vi "Insert Loop.vi"(4 "Loop Iterations":i32, 6 "Insertion Index":i32=-1, 7 "Parent ID":string, 8 "error in (no error)":errorcluster, 9 "Unique ID":string, 10 "Name":string, 11 "Custom Type Test Executive in":refnum<class "Custom Type Test Executive.lvclass">) -> (0 "error out":errorcluster, 1 "Replaced?":bool, 2 "Unique ID out":string, 3 "Custom Type Test Executive out":refnum<class "Custom Type Test Executive.lvclass">)   [LabVIEW 2017, in "Custom Type Test Executive.lvlib" / "Custom Type Test Executive.lvclass"]
uses:
  <vilib>/gpm_packages/@cs/test-executive/Source/Custom Type Test Executive/Custom Type Test Executive/Custom Type Test Executive.lvclass
  C:/Program Files/National Instruments/LabVIEW 2017/vi.lib/gpm_packages/@cs/test-executive/Source/Test Executive/TestExecutive/Test Executive.lvclass
  <vilib>/gpm_packages/@cs/test-executive/Source/Custom Type Test Executive/Loop/Loop.lvclass
  <vilib>/gpm_packages/@cs/data-type-serializer/source/Boolean/Boolean.lvclass/Boolean.ctl
  <vilib>/gpm_packages/@cs/data-type-serializer/source/I32/I32.lvclass/I32.ctl
  <vilib>/gpm_packages/@cs/test-executive/Source/Test Executive/TestExecutive/Test Executive.lvclass/Test Executive.ctl
  eff3c389-d19d-4e12-abfe-b5bcb03aec03.vi
  3b5f5b1c-5d92-47fe-9b34-6cf7948e1255.vi
  2e520cd6-f760-4b31-8e6b-f4272244ae2a.vi
  34c56a90-4072-42ae-b3b1-584153b934c7.vi
  <vilib>/gpm_packages/@cs/data-type-serializer/source/I32/I32.lvclass
  <vilib>/gpm_packages/@cs/data-type-serializer/source/Boolean/Boolean.lvclass
  <vilib>/gpm_packages/@cs/linked-list/Source/Linked List/ILinkedList/ILinked List.lvclass
  <vilib>/gpm_packages/@cs/linked-list/Source/Linked List/Linked List Ref/Linked List Ref.lvclass
  <vilib>/gpm_packages/@cs/test-executive/Source/Test Executive/TestExecutive/Test Executive.lvclass
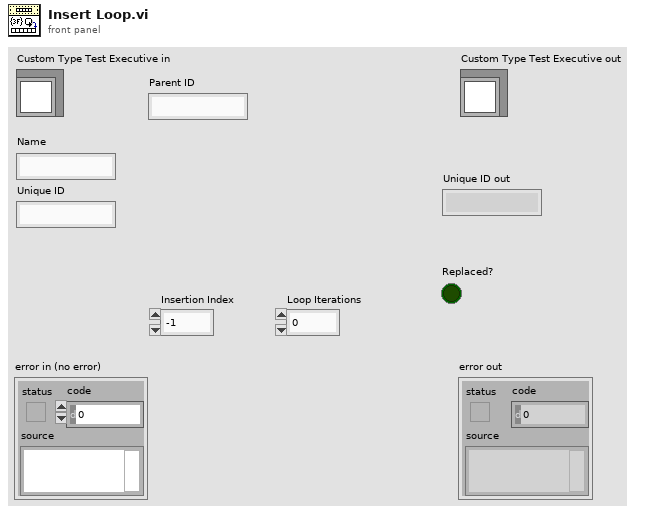
[diagram p1: front panel]
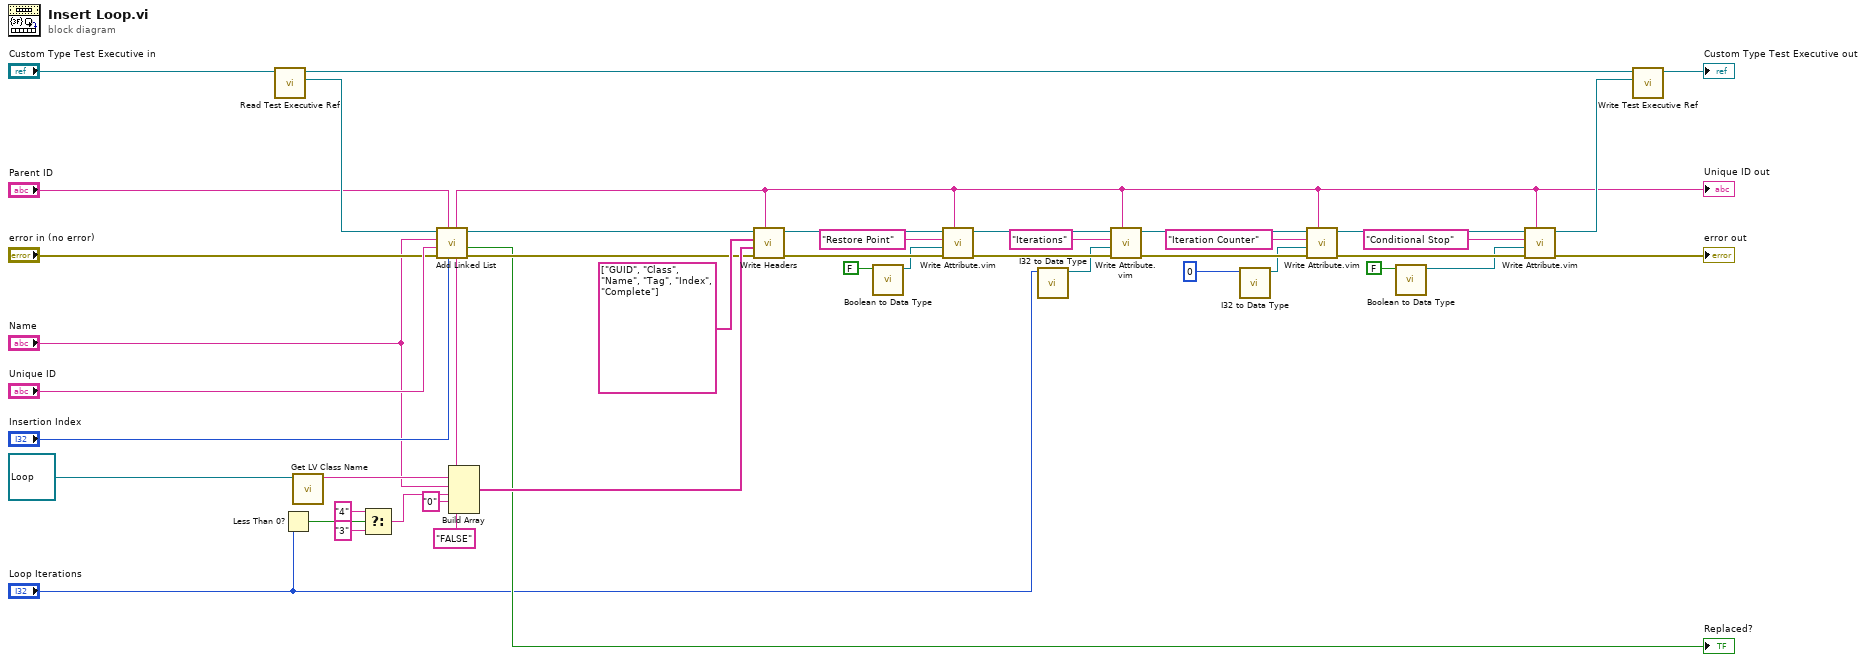
[diagram p0: block diagram]
diagram:
  n1 = call <vilib>:"Read Test Executive Ref.vi"("Test Executive in"="Custom Type Test Executive in") -> ("Test Executive Ref"=w21:refnum<data-value>, "Test Executive out"=w20:refnum<class "Custom Type Test Executive.lvclass">)  [unwired: 9 in]
  n2 = Less Than 0?(x="Loop Iterations") -> (x < 0?=w37:bool)
  n3 = call <vilib>:"Get LV Class Name.vi"("object"=refnum<class "Loop.lvclass"> refnum ("Custom Type Test Executive.lvlib:Loop.lvclass")) -> ("class name"=w41:string)  [unwired: 9 in, 1 out]
  n4 = Select(t="4" ("Tag"), s=w37, f="3" ("Tag")) -> (s? t:f=w34:string)
  n5 = call <vilib>:"Add Linked List.vi"("Insertion Index"="Insertion Index", "Parent ID"="Parent ID", "error in (no error)"="error in (no error)", "Linked List ID"="Unique ID", "Name"="Name", "Linked List Ref"=w21) -> ("error out"=w42:errorcluster, "Replaced?"=→"Replaced?":bool, "Linked List Ref out"=w43:refnum<data-value>, "Linked List ID out"=w12:string)  [unwired: 2 in]
  "Unique ID out" <- w12
  n6 = Build Array(w12, w41, "Name", w34, "0" ("element"), "FALSE" ("element")) -> (w44:string[])
  n7 = call <vilib>:"Write Headers.vi"("Linked List ID"=w12, "error in (no error)"=w42, "Header Values"=w44, "Header Names"=string[] ["GUID", "Class", "Name", "Tag", "Index", "Complete"], "Linked List Ref"=w43) -> ("error out"=w38:errorcluster, "Linked List Ref out"=w39:refnum<data-value>)  [unwired: 5 in]
  n8 = call <vilib>:"Boolean to Data Type.vi"("Boolean"=FALSE) -> ("Boolean out"=w7:refnum<class "Boolean.lvclass">)  [unwired: 9 in, 1 out]
  n9 = call "Write Attribute.vim"("Linked List ID"=w12, "error in (no error)"=w38, "Attribute"=w7, "Attribute Name"="Restore Point", "Linked List Ref"=w39) -> ("error out"=w27:errorcluster, "Linked List Ref out"=w30:refnum<data-value>)  [unwired: 3 in, 2 out]
  n10 = call <vilib>:"I32 to Data Type.vi"("I32"="Loop Iterations") -> ("Boolean out"=w5:refnum<class "I32.lvclass">)  [unwired: 9 in, 1 out]
  n11 = call "Write Attribute.vim"("Linked List ID"=w12, "error in (no error)"=w27, "Attribute"=w5, "Attribute Name"="Iterations", "Linked List Ref"=w30) -> ("error out"=w26:errorcluster, "Linked List Ref out"=w29:refnum<data-value>)  [unwired: 3 in, 2 out]
  n12 = call <vilib>:"I32 to Data Type.vi"("I32"=0 ("Numeric")) -> ("Boolean out"=w3:refnum<class "I32.lvclass">)  [unwired: 9 in, 1 out]
  n13 = call "Write Attribute.vim"("Linked List ID"=w12, "error in (no error)"=w26, "Attribute"=w3, "Attribute Name"="Iteration Counter", "Linked List Ref"=w29) -> ("error out"=w25:errorcluster, "Linked List Ref out"=w28:refnum<data-value>)  [unwired: 3 in, 2 out]
  n14 = call <vilib>:"Boolean to Data Type.vi"("Boolean"=FALSE) -> ("Boolean out"=w1:refnum<class "Boolean.lvclass">)  [unwired: 9 in, 1 out]
  n15 = call "Write Attribute.vim"("Linked List ID"=w12, "error in (no error)"=w25, "Attribute"=w1, "Attribute Name"="Conditional Stop", "Linked List Ref"=w28) -> ("error out"=→"error out":errorcluster, "Linked List Ref out"=w18:refnum<data-value>)  [unwired: 3 in, 2 out]
  n16 = call <vilib>:"Write Test Executive Ref.vi"("Test Executive Ref"=w18, "Test Executive in"=w20) -> ("Test Executive out"=→"Custom Type Test Executive out":refnum<class "Custom Type Test Executive.lvclass">)  [unwired: 9 in]
